vi "GPS Tester.vi"() -> ()   [LabVIEW 2010]
uses:
  New Sensor Drivers/Novatel GPS new.llb/GPSINS output.ctl
panel:
  in  "Array":dbl[](array[numeric])
  in  "OK Button":bool
  in  "Tab Control":enum32{"Page 1", "Page 2"}(tab)
  out "GPS cluster":T1 {"Northing" format="%#.2f"; "Easting" format="%#.2f"}
  in  "GPS Com":refnum<visa-resource-name>
  out "GPS Data":T2 {"Easting" format="%#.10f"; "Northing" format="%#.10f"}
  in  "stop":bool
  out "GPS Status":T3
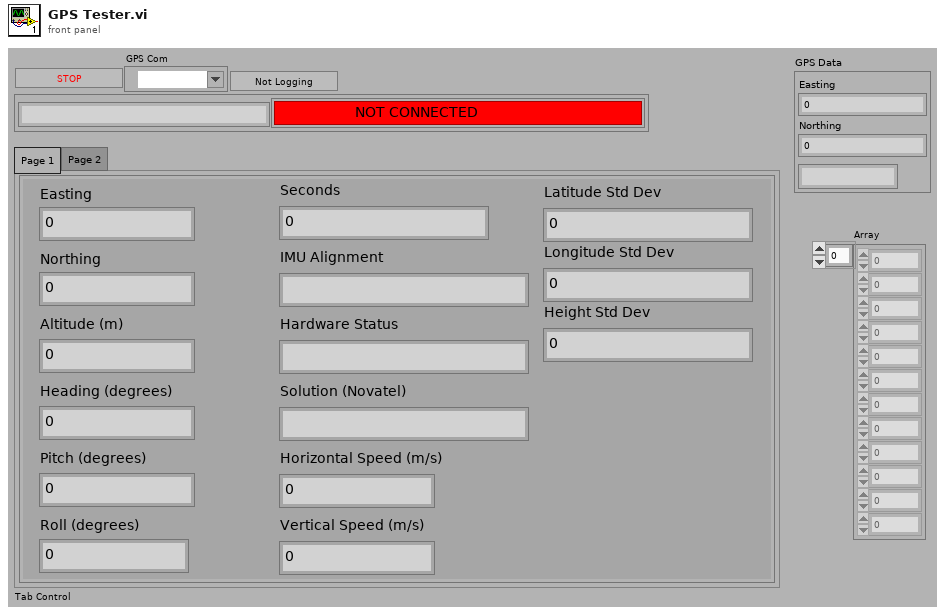
[diagram p1: front panel]
types:
  T1 = typedef "GPSINS output.ctl" = cluster{"Easting ":dbl, "Northing":dbl, "Horizontal Speed (m/s)":dbl, "Heading (degrees)":dbl, "Pitch (degrees)":dbl, "Roll (degrees)":dbl, "IMU Alignment":string, "Hardware Status":string, "Solution (Novatel)":string, "Altitude (m)":dbl, "Vertical Speed (m/s)":dbl, "Seconds":u32, "Latitude Std Dev":dbl, "Longitude Std Dev":dbl, "Height Std Dev":dbl}
  T2 = cluster{"Easting":dbl, "Northing":dbl, "Status":string}
  T3 = cluster{"GPS Connected":bool, "GPS Connect Status":string}
  T4 = enum16{"open", "replace", "create", "open or create", "replace or create", "replace or create with confirmation"}
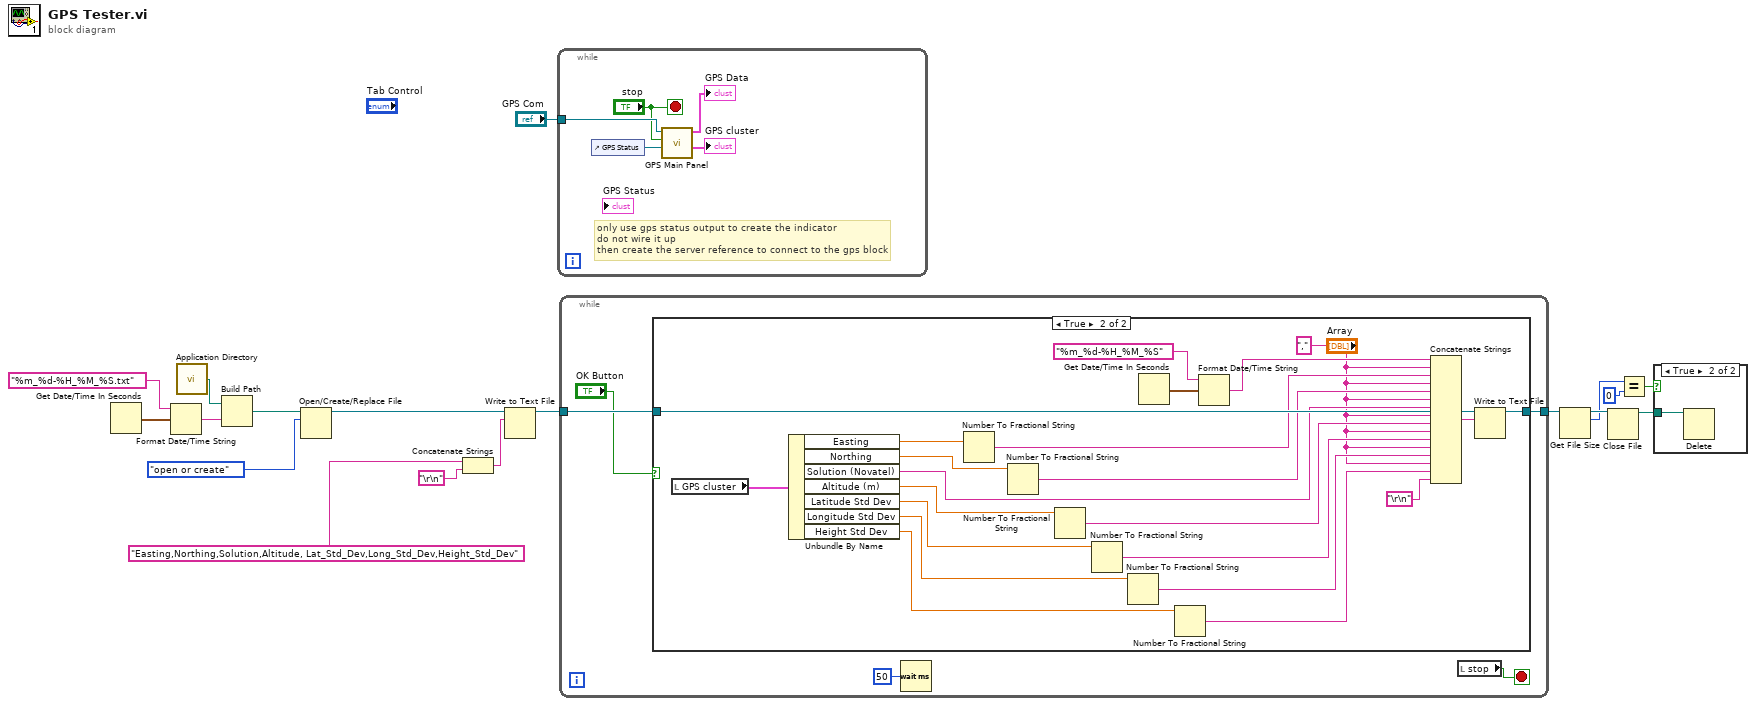
[diagram p0: block diagram]
diagram:
  n1 = Get Date/Time In Seconds() -> (seconds since 1Jan1904=w10:timestamp)
  n2 = Format Date/Time String(time format string (%c)="%m_%d-%H_%M_%S.txt", seconds (now)=w10) -> (date/time string=w8:string)  [unwired: 1 in]
  n3 = call <vilib>:"Application Directory.vi"() -> ("Application Directory"=w17:path)
  n4 = Build Path(base path=w17, name or relative path=w8) -> (appended path=w16:path)
  n5 = Open/Create/Replace File(file path (use dialog)=w16, operation (0:open)=T4."open or create") -> (refnum out=w7:refnum<file>)  [unwired: 4 in, 2 out]
  n6 = Concatenate Strings("Easting,Northing,Solution,Altitude, Lat_Std_Dev,Long_Std_Dev,Height_Std_Dev", "\r\n") -> (w3:string)
  n7 = Write to Text File(file (use dialog)=w7, text=w3) -> (refnum out=w6:refnum<file>)  [unwired: 2 in, 2 out]
  n8 = while {
    tunnel: "GPS Com" -> [w23]
    stop <- "stop" stop-if-true
    # "only use gps status output to create the indicator\ndo not wire it up\nthen create the server reference to connect to the gps block"
    n9 = control-ref of="GPS Status"() -> (w19:refnum<vi>)
    n10 = call "GPS Main Panel.vi"("GPS Com"=w23, "stop"="stop", "GPS Status Ref"=w19) -> ("GPS Data"=→"GPS Data":T2, "GPS cluster"=→"GPS cluster":T1)  [unwired: 3 in, 2 out]
  }
  n11 = while {
    tunnel: w6 -> [w27]
    tunnel: [w25] -> w12
    stop <- w28 stop-if-true
    n12 = case shown="True" "OK Button" {
      tunnel: w27 -> [w29 w51]
      tunnel: [w29 w50] -> w25
      frame False {
      }
      frame True {
        w33 = ","
        n13 = local read "GPS cluster"() -> (w49:T1)
        n14 = Unbundle By Name(w49) -> ("Easting"=w48:dbl, "Northing"=w42:dbl, "Solution (Novatel)"=w40:string, "Altitude (m)"=w39:dbl, "Latitude Std Dev"=w37:dbl, "Longitude Std Dev"=w35:dbl, "Height Std Dev"=w32:dbl)
        n15 = Number To Fractional String(number=w48) -> (F-format string=w43:string)  [unwired: 3 in]
        n16 = Number To Fractional String(number=w42) -> (F-format string=w41:string)  [unwired: 3 in]
        n17 = Number To Fractional String(number=w39) -> (F-format string=w38:string)  [unwired: 3 in]
        n18 = Number To Fractional String(number=w37) -> (F-format string=w36:string)  [unwired: 3 in]
        n19 = Number To Fractional String(number=w35) -> (F-format string=w34:string)  [unwired: 3 in]
        n20 = Get Date/Time In Seconds() -> (seconds since 1Jan1904=w45:timestamp)
        n21 = Number To Fractional String(number=w32) -> (F-format string=w31:string)  [unwired: 3 in]
        n22 = Format Date/Time String(time format string (%c)="%m_%d-%H_%M_%S", seconds (now)=w45) -> (date/time string=w44:string)  [unwired: 1 in]
        n23 = Concatenate Strings(w44, w33, w43, w33, w41, w33, w40, w33, w38, w33, w36, w33, w34, w33, w31, "\r\n") -> (w47:string)
        n24 = Write to Text File(file (use dialog)=w51, text=w47) -> (refnum out=w50:refnum<file>)  [unwired: 2 in, 2 out]
      }
    }
    n25 = Wait (ms)(milliseconds to wait=u32 50) -> ()  [unwired: 1 out]
    n26 = local read "stop"() -> (w28:bool)
  }
  n27 = Get File Size(file=w12) -> (refnum out=w13:refnum<file>, size (in bytes)=w2:i64)  [unwired: 1 in, 1 out]
  n28 = Close File(refnum=w13) -> (path=w14:path)  [unwired: 1 in, 1 out]
  n29 = Equal?(x=w2, y=i64 0) -> (x = y?=w11:bool)
  n30 = case shown="True" w11 {
    tunnel: w14 -> [_ w52]
    frame False {
    }
    frame True {
      n31 = Delete(path (use dialog)=w52) -> ()  [unwired: 4 in, 3 out]
    }
  }
